vi "3b - QDSM message as class.vi"() -> ()   [LabVIEW 2015]
uses:
  State/Parent Actor.lvclass
  Parent Message/Parent Message.lvclass
  Turn On/Turn On.lvclass
  Child Actor/Child Actor.lvclass
  Toggle/Toggle.lvclass
panel:
  in  "Choose Actor":bool
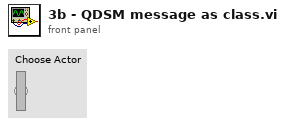
[diagram p1: front panel]
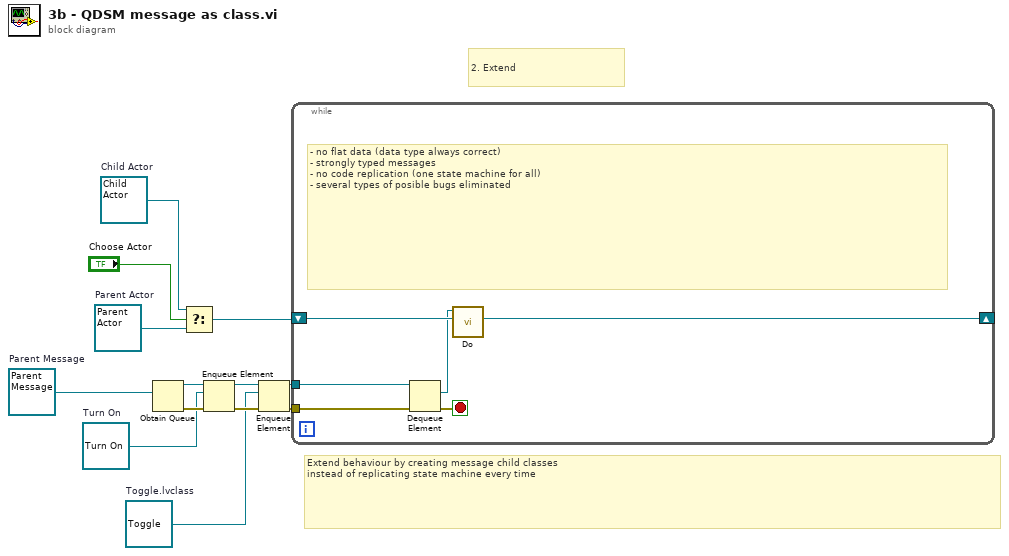
[diagram p0: block diagram]
diagram:
  w1 = refnum<class "Toggle.lvclass"> refnum  # Toggle.lvclass
  w3 = refnum<class "Child Actor.lvclass"> refnum  # Child Actor
  w4 = refnum<class "Turn On.lvclass"> refnum  # Turn On
  w5 = refnum<class "Parent Message.lvclass"> refnum  # Parent Message
  w7 = refnum<class "Parent Actor.lvclass"> refnum  # Parent Actor
  # "2. Extend"
  # "Extend behaviour by creating message child classes\ninstead of replicating state machine every time"
  n1 = Obtain Queue(element data type=w5) -> (queue out=w9:refnum<queue>, error out=w11:errorcluster)  [unwired: 4 in, 1 out]
  n2 = Select(t=w3, s="Choose Actor", f=w7) -> (s? t:f=w6:refnum<class "Parent Actor.lvclass">)
  n3 = Enqueue Element(queue=w9, element=w4, error in (no error)=w11) -> (queue out=w8:refnum<queue>, error out=w10:errorcluster)  [unwired: 1 in, 1 out]
  n4 = Enqueue Element(queue=w8, element=w1, error in (no error)=w10) -> (queue out=w12:refnum<queue>, error out=w13:errorcluster)  [unwired: 1 in, 1 out]
  n5 = while {
    tunnel: w13 -> [w19]
    tunnel: w12 -> [w18]
    shift-right: [w14] -> _
    shift-left: w6 -> [w16]
    stop <- w17 stop-if-true
    # "- no flat data (data type always correct)\n- strongly typed messages\n- no code replication (one state machine for all)\n- several types of posible bugs eliminated"
    n6 = Dequeue Element(queue=w18, error in (no error)=w19) -> (element=w15:refnum<class "Parent Message.lvclass">, error out=w17:errorcluster)  [unwired: 1 in, 2 out]
    n7 = call-dynamic "Do.vi"("Parent Actor"=w16, "Parent Message in"=w15) -> ("Parent Actor out"=w14:refnum<class "Parent Actor.lvclass">)  [unwired: 7 in, 2 out]
  }
